vi "CRYAcq Save to Curve.vi"(0 "Acquisition Type":u16, 1 "Setup in":T1={"No.VI"=0, "Category"="", "StepName"="", "Seq setup flattened"="", "Comment"="", "Steps config."=[], "Jump config"=[], "Start"=0.0, "Increment"=0.0, "Name"="Pa", "Unit"="Pa", "Y data"=1, "Y prefix"="", "Y dB ref"=1.0, "Y unit"="", "Repeat State Array"=[]} {"Repeat State Array"."Start" format="%#_5g"; "Y dB ref" format="%.1f"; "Y data" items=["dB", "Lin"]; "Start" format="%#_5g"}, 5 "Data In":T5[](array[typedef]) {"Z data" items=["dB", "Lin"]; "X data" items=["dB", "Lin"]; "Y data" items=["dB", "Lin"]; "Z dB ref" format="%.1f"; "Z axis" items=["Log", "Lin"]; "X dB ref" format="%.1f"; "X axis" items=["Log", "Lin"]; "Y axis" items=["Log", "Lin"]; "Y dB ref" format="%.1f"; "Curve"."z" format="%.2f"; "Curve"."y" format="%.2f"; "Curve"."x" format="%.2f"}, 9 "Wave In":T2 {"Y dB ref" format="%.1f"; "Y axis" items=["Log", "Lin"]; "Y data" items=["dB", "Lin"]; "X data" items=["dB", "Lin"]}, 11 "Is Save?":bool) -> (4 "Inserted Names Out":string[](array[string]))   [LabVIEW 2013]
uses:
  Typedef Control/CRYData Cluster.ctl
  Typedef Control/CRYWaveform Cluster Array.ctl
  Typedef Control/CRYWaveform Cluster.ctl
  Typedef Control/CRYData Variant Array.ctl
  Typedef Control/CRYStep.ctl
  Task Sequence/CRYProject Run Control Global.vi
panel:
  out "Wave In Indicater":T2 {"Y dB ref" format="%.1f"; "Y axis" items=["Log", "Lin"]; "Y data" items=["dB", "Lin"]; "X data" items=["dB", "Lin"]}
  in  "Data":T4
  # "0-Play & Record\n1-Record\n2-Sine Generator\n3-Voltmeter\n4-Oscilloscope\n5-Spectrum Analyzer\n6-RTA\n7-Generator & Voltmeter\n8-Generator & Oscilloscope\n9-Generator & Spectrum\n10-Generator & RTA\n11-Read From DC Connect"
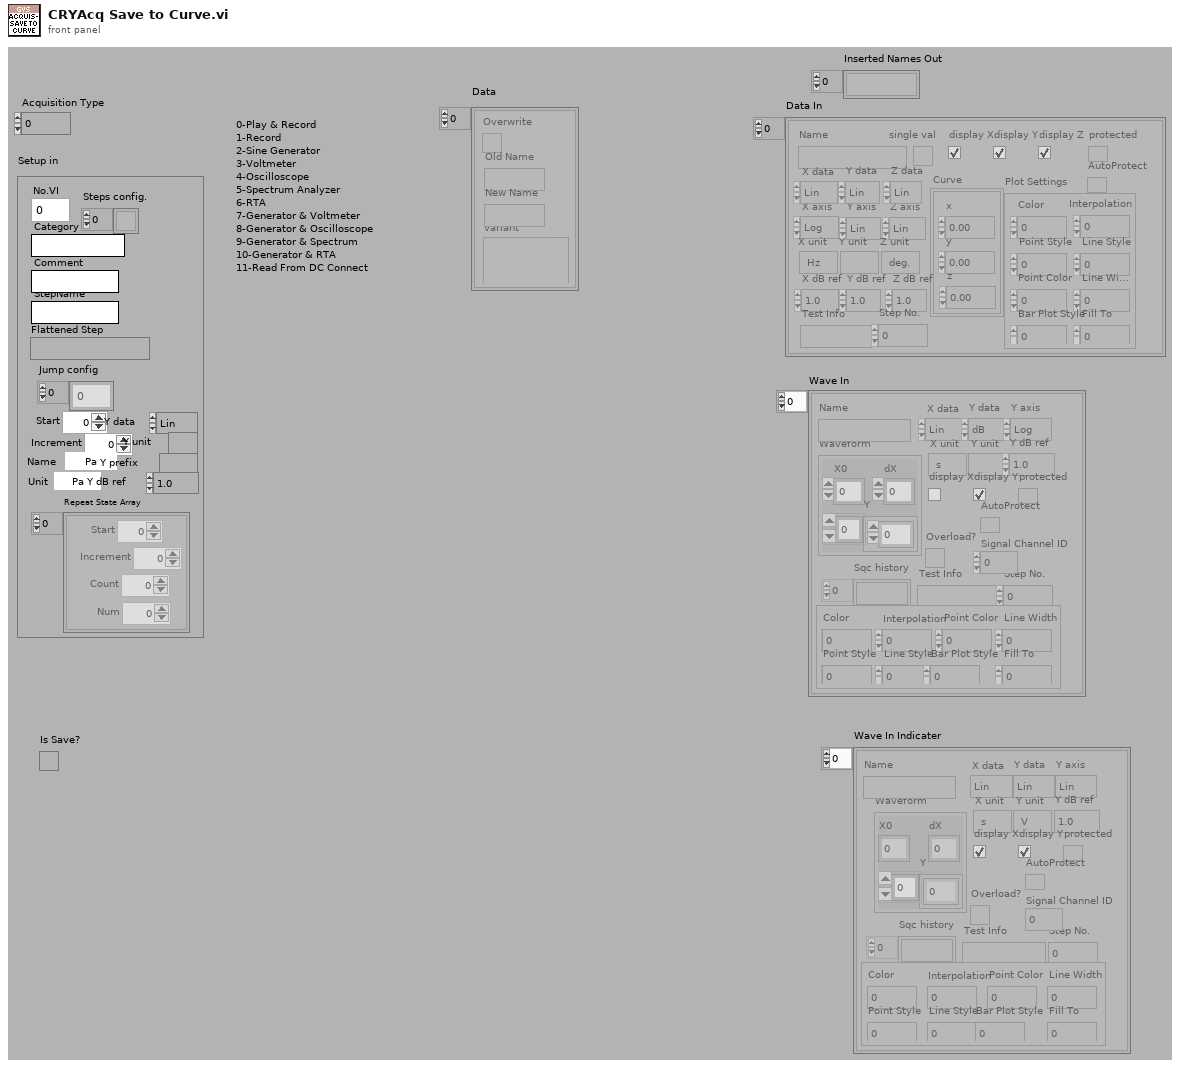
[diagram p1: front panel]
types:
  T1 = typedef "CRYStep.ctl" = cluster{"No.VI":i32, "Category":string, "StepName":string, "Seq setup flattened":string, "Comment":string, "Steps config.":bool[], "Jump config":i32[], "Start":dbl, "Increment":dbl, "Name":string, "Unit":string, "Y data":u16, "Y prefix":string, "Y dB ref":dbl, "Y unit":string, "Repeat State Array":cluster{"Start":dbl, "Increment":dbl, "Count":i32, "Num":i32}[]}
  T2 = typedef "CRYWaveform Cluster Array.ctl" = T3[]
  T3 = typedef "CRYWaveform Cluster.ctl" = cluster{"Waveform":cluster{"X0":dbl, "dX":dbl, "Y":sgl[]}, "X data":u16, "Y data":u16, "Y axis":u16, "X unit":string, "Y unit":string, "Y dB ref":dbl, "display Y":bool, "display X":bool, "Overload?":bool, "Test Info":string, "Step No.":i32, "Name":string, "protected":bool, "Sqc history":string[], "Signal Channel ID":i32, "Plot Settings":cluster{"Color":u32, "Interpolation":u8, "Point Style":u8, "Line Style":u8, "Point Color":u32, "Line Width":u8, "Bar Plot Style":u8, "Fill To":i16}, "AutoProtect":bool}
  T4 = typedef "CRYData Variant Array.ctl" = cluster{"variant":variant, "Overwrite":bool, "Old Name":string, "New Name":string}[]
  T5 = typedef "CRYData Cluster.ctl" = cluster{"Name":string, "Curve":cluster{"x":dbl, "y":dbl, "z":dbl}[], "X data":u16, "Y data":u16, "Z data":u16, "X axis":u16, "Y axis":u16, "Z axis":u16, "X unit":string, "Y unit":string, "Z unit":string, "X dB ref":dbl, "Y dB ref":dbl, "Z dB ref":dbl, "single val":bool, "protected":bool, "display X":bool, "display Y":bool, "display Z":bool, "Test Info":string, "Step No.":i32, "Plot Settings":cluster{"Color":u32, "Interpolation":u8, "Point Style":u8, "Line Style":u8, "Point Color":u32, "Line Width":u8, "Bar Plot Style":u8, "Fill To":i16}, "AutoProtect":bool}
  T6 = cluster{"Start":dbl, "Increment":dbl, "Count":i32, "Num":i32}[]
  T7 = cluster{"Color":u32, "Interpolation":u8, "Point Style":u8, "Line Style":u8, "Point Color":u32, "Line Width":u8, "Bar Plot Style":u8, "Fill To":i16}
  T8 = typedef "CRYData Cluster Array.ctl" = T5[]
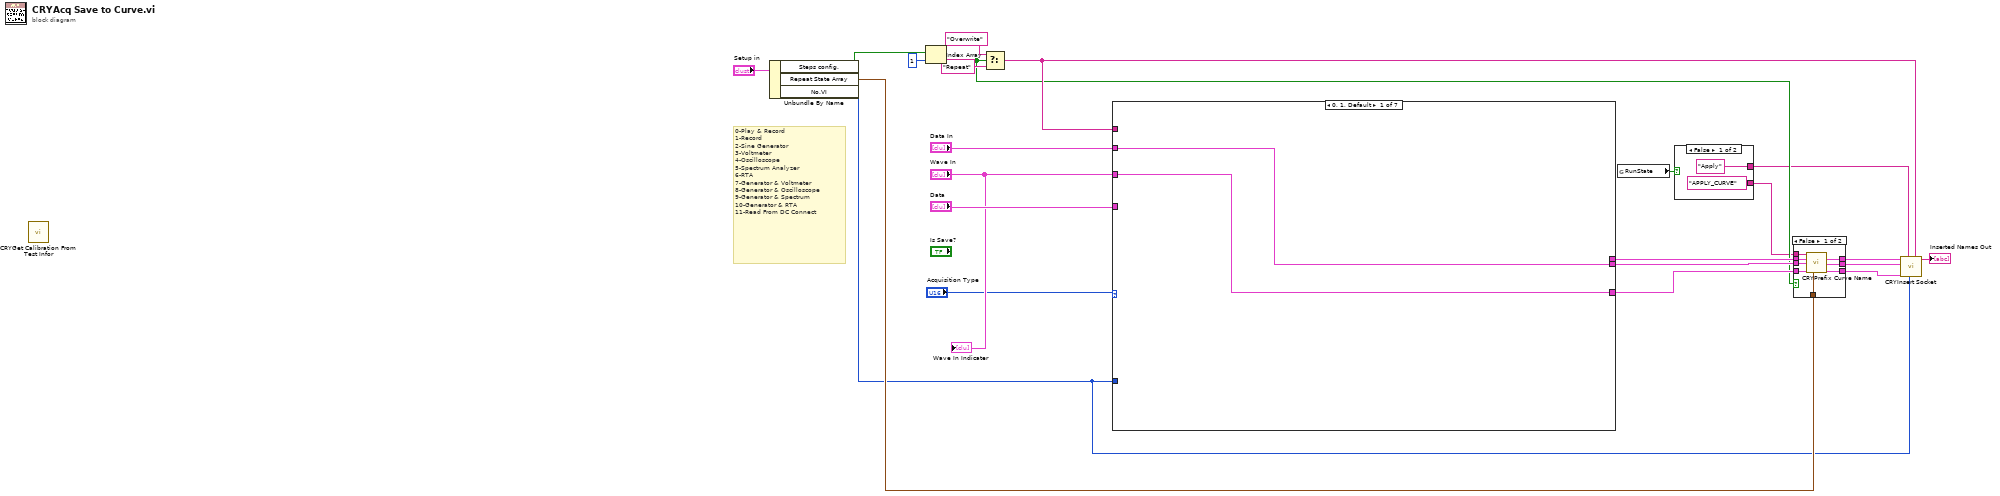
[diagram p0: block diagram]
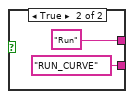
[diagram p2: hidden frame]
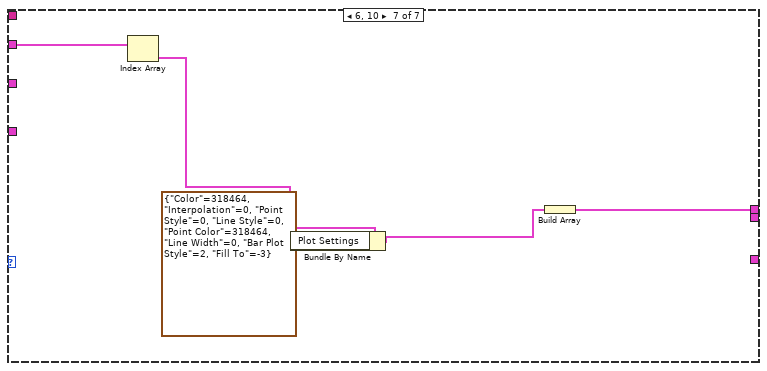
[diagram p9: hidden frame]
diagram:
  # "0-Play & Record\n1-Record\n2-Sine Generator\n3-Voltmeter\n4-Oscilloscope\n5-Spectrum Analyzer\n6-RTA\n7-Generator & Voltmeter\n8-Generator & Oscilloscope\n9-Generator & Spectrum\n10-Generator & RTA\n11-Read From DC Connect"
  n1 = call "CRYGet Calibration From Test Infor.vi"() -> ()  [unwired: 7 in, 5 out]
  n2 = Unbundle By Name("Setup in") -> ("Steps config."=w9:bool[], "Repeat State Array"=w8:T6, "No.VI"=w7:i32)
  n3 = Index Array(array=w9, index=1) -> (element=w11:bool)
  n4 = Select(t="Overwrite" ("Y unit"), s=w11, f="Repeat") -> (s? t:f=w18:string)
  n5 = case shown="0, 1, Default" "Acquisition Type" {
    tunnel: "Wave In" -> [w25 w26 _ _ w29 _ _]
    tunnel: "Data" -> [_ _ _ _ _ _ _]
    tunnel: "Data In" -> [w24 _ _ w27 w28 w30 w35]
    tunnel: w7 -> [_ _ _ _ _ _ _]
    tunnel: w18 -> [_ _ _ _ _ _ _]
    tunnel: [_ _ _ _ _ w30 w31] -> w17
    tunnel: [w25 w26 _ _ w29 _ _] -> w15
    tunnel: [w24 _ _ w27 w28 _ _] -> w16
    frame 0, 1, Default {
    }
    frame 11 {
    }
    frame 2 {
    }
    frame 3, 7 {
    }
    frame 4, 8 {
    }
    frame 5, 9 {
    }
    frame 6, 10 {
      n6 = Index Array(array=w35) -> (element=w34:T5)  [unwired: 1 in]
      n7 = Bundle By Name(cluster=w34, "Plot Settings"=T7 {"Color"=318464, "Interpolation"=0, "Point Style"=0, "Line Style"=0, "Point Color"=318464, "Line Width"=0, "Bar Plot Style"=2, "Fill To"=-3}) -> (w32:T5)
      n8 = Build Array(w32) -> (w31:T5[])
    }
  }
  n9 = global read "CRYProject Run Control Global.vi" "RunState"() -> (w6:bool)
  n10 = case shown="False" w6 {
    tunnel: ["Apply" ("sOption1") "Run" ("Type In")] -> w5
    tunnel: ["APPLY_CURVE" ("Type In") "RUN_CURVE" ("Type In")] -> w4
    frame False {
    }
    frame True {
    }
  }
  n11 = case shown="False" w11 {
    tunnel: w4 -> [w47 _]
    tunnel: w17 -> [w46 w50]
    tunnel: w16 -> [w45 w49]
    tunnel: w15 -> [w44 w48]
    tunnel: [w43 w48] -> w14
    tunnel: [w42 w49] -> w13
    tunnel: [w41 w50] -> w12
    tunnel: w8 -> [w40 _]
    frame False {
      n12 = call "CRYPrefix Curve Name.vi"("Type In"=w47, "Curves In"=w46, "Values In"=w45, "Waves In"=w44, "Repeat State Array In"=w40) -> ("Curves Out"=w41:T8, "Values Out"=w42:T8, "Waves Out"=w43:T2)  [unwired: 7 in, 1 out]
    }
    frame True {
    }
  }
  n13 = call "CRYInsert Socket.vi"("sOption2"=w18, "Step No."=w7, "sOption1"=w5, "Waves"=w14, "Values"=w13, "Curves"=w12) -> ("Inserted Names Out"=→"Inserted Names Out":string[])  [unwired: 5 in]
  "Wave In Indicater" <- "Wave In"
